vi "Acquire.vi"(8 "error in (no error)":errorcluster, 9 "Data Queue":refnum<queue>, 10 "Data Notifier":refnum<notifier>, 11 "Hardware Resources in":T1) -> (0 "error out":errorcluster, 3 "Hardware Resources out":T1)   [LabVIEW 2013, in "Acquisition.lvlib"]
doc: "Perform the acquisition. Replace the contents of this diagram with calls to acquisition hardware."
uses:
  Acquisition.lvlib
  Hardware Configuration.ctl
  C:/Program Files (x86)/National Instruments/LabVIEW 2013/vi.lib/ULx/ULx_LV.dll
  <vilib>/ULx/Read.llb/ULx Read (Analog 1D Wfm NChan NSamp).vi
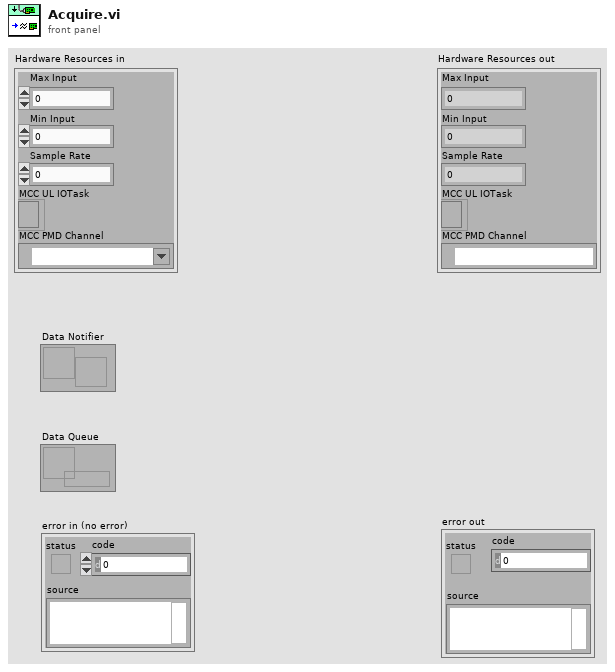
[diagram p1: front panel]
types:
  T1 = typedef "Acquisition.lvlib/Hardware Configuration.ctl" = cluster{"Max Input":dbl, "Min Input":dbl, "Sample Rate":dbl, "MCC UL IOTask":refnum<k24>, "MCC PMD Channel":refnum<k21>}
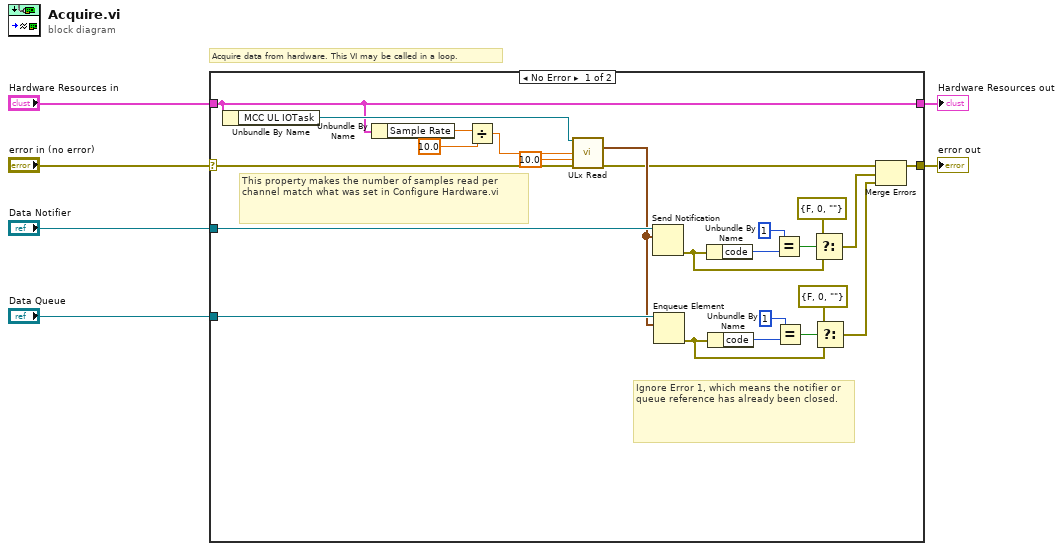
[diagram p0: block diagram]
diagram:
  # "Acquire data from hardware. This VI may be called in a loop."
  n1 = case shown="No Error" "error in (no error)" {
    selector: "error in (no error)" -> [w11 w31]
    tunnel: [w30 w31] -> w5
    tunnel: "Hardware Resources in" -> [w9 w32]
    tunnel: [w9 w32] -> w3
    tunnel: "Data Notifier" -> [w29 _]
    tunnel: "Data Queue" -> [w16 _]
    frame No Error {
      # "This property makes the number of samples read per channel match what was set in Configure Hardware.vi"
      # "Ignore Error 1, which means the notifier or queue reference has already been closed."
      n2 = Unbundle By Name(w9) -> ("MCC UL IOTask"=w14:refnum<k24>)
      n3 = Unbundle By Name(w9) -> ("Sample Rate"=w13:dbl)
      n4 = Divide(x=w13, y=10.0) -> (x/y=w12:dbl)
      n5 = call-poly <vilib>:"ULx Read.vi"("task in"=w14, "number of samples per channel"=w12, "timeout"=10.0, "error in"=w11) -> ("data"=w15:waveform(dbl)[], "error out"=w7:errorcluster)  [unwired: 9 in, 1 out]
      n6 = Send Notification(notification=w15, notifier=w29) -> (error out=w25:errorcluster)  [unwired: 1 in, 1 out]
      n7 = Enqueue Element(queue=w16, element=w15) -> (error out=w21:errorcluster)  [unwired: 2 in, 2 out]
      n8 = Unbundle By Name(w25) -> ("code"=w28:i32)
      n9 = Unbundle By Name(w21) -> ("code"=w18:i32)
      n10 = Equal?(x=1, y=w28) -> (x = y?=w26:bool)
      n11 = Equal?(x=1, y=w18) -> (x = y?=w20:bool)
      n12 = Select(t=errorcluster {"status"=FALSE, "code"=0, "source"=""} ("error constant"), s=w26, f=w25) -> (s? t:f=w24:errorcluster)
      n13 = Select(t=errorcluster {"status"=FALSE, "code"=0, "source"=""} ("error constant"), s=w20, f=w21) -> (s? t:f=w17:errorcluster)
      n14 = Merge Errors(w7, w24, w17) -> (w30:errorcluster)
    }
    frame Error {
    }
  }
  "Hardware Resources out" <- w3
  "error out" <- w5
